vi "GEOM_Coords2Size.vi"(10 "Coords":T2) -> (2 "Size":T1)   [LabVIEW 2016]
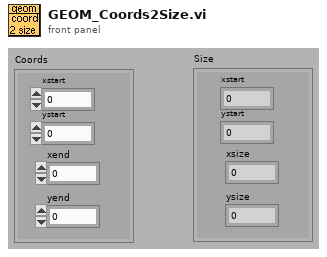
[diagram p1: front panel]
types:
  T1 = cluster{"xstart":i32, "ystart":i32, "xsize":i32, "ysize":i32}
  T2 = cluster{"xstart":i32, "ystart":i32, "xend":i32, "yend":i32}
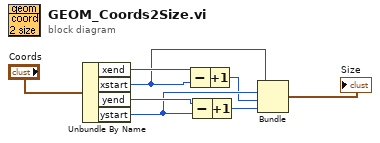
[diagram p0: block diagram]
diagram:
  n1 = Unbundle By Name("Coords") -> ("xend"=w9:i32, "xstart"=w7:i32, "yend"=w8:i32, "ystart"=w6:i32)
  n2 = Subtract(x=w9, y=w7) -> (x-y=w5:i32)
  n3 = Subtract(x=w8, y=w6) -> (x-y=w4:i32)
  n4 = Increment(x=w5) -> (x+1=w3:i32)
  n5 = Increment(x=w4) -> (x+1=w2:i32)
  n6 = Bundle("xstart"=w7, "ystart"=w6, w3, w2) -> (→"Size":cluster{"xstart":i32, "ystart":i32, i32, i32})  [unwired: 1 out]
